vi "Define Parameter.vi"(8 "error in (no error)":errorcluster, 11 "Analyze Distanz in":refnum<class "Analyze Distanz.lvclass">) -> (0 "error out":errorcluster, 3 "Analyze Distanz out":refnum<class "Analyze Distanz.lvclass">)   [LabVIEW 2014, in "Analyze.lvlib" / "Analyze Distanz.lvclass"]
uses:
  Analyze Distanz.lvclass
  Analyze BaseClass/Analyze BaseClass/Analyze BaseClass.lvclass
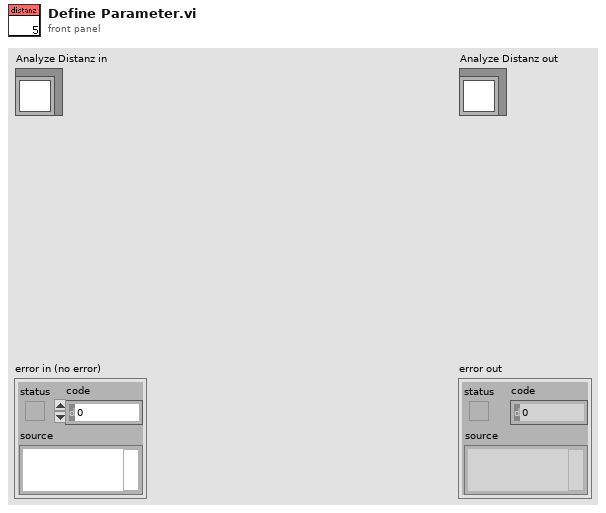
[diagram p1: front panel]
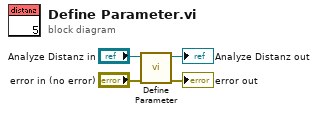
[diagram p0: block diagram]
diagram:
  n1 = call-parent "Define Parameter.vi"("error in (no error)"="error in (no error)", "Analyze BaseClass in"="Analyze Distanz in") -> ("error out"=→"error out":errorcluster, "Analyze BaseClass out"=→"Analyze Distanz out":refnum<class "Analyze Distanz.lvclass">)  [unwired: 8 in]
